vi "Validate Sequence File.vi"(8 "error in (no error)":errorcluster, 11 "Configured Steps In":T1[](array[typedef])) -> (0 "error out":errorcluster, 2 "Valid?":bool, 3 "Configured Steps Out":T1[](array[typedef]))   [LabVIEW 2018]
doc: "Compares the step names from the saved sequence file with the available steps. If one does not match, returns error 71."
uses:
  controls/Configured Step.ctl
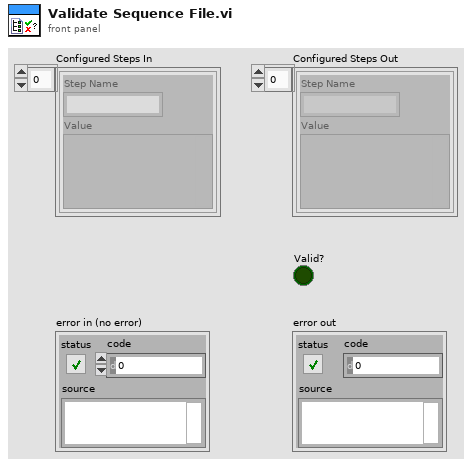
[diagram p1: front panel]
types:
  T1 = typedef "Configured Step.ctl" = cluster{"Step Name":string, "Value":variant}
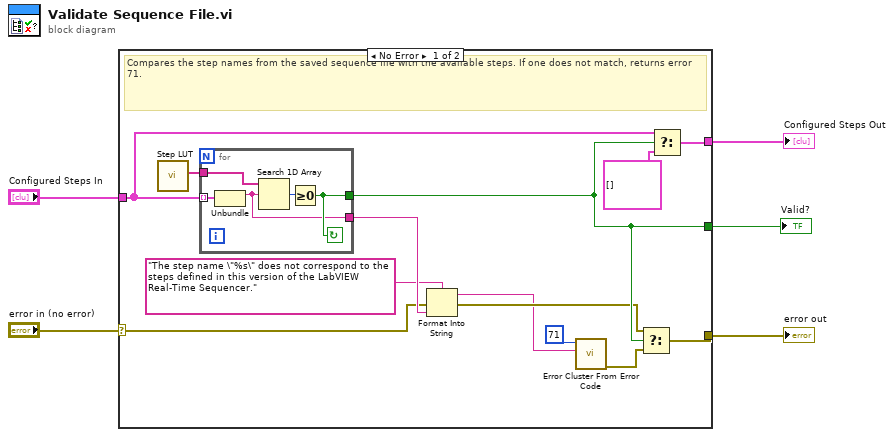
[diagram p0: block diagram]
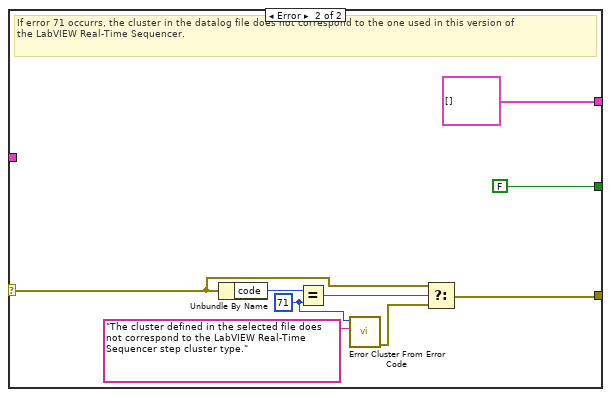
[diagram p2: hidden frame]
diagram:
  n1 = case shown="No Error" "error in (no error)" {
    selector: "error in (no error)" -> [w9 w25]
    tunnel: "Configured Steps In" -> [w14 _]
    tunnel: [w17 T1[] [] ("Configured Steps In")] -> w5
    tunnel: [w15 w24] -> w2
    tunnel: [w16 FALSE] -> w1
    frame No Error {
      # "Compares the step names from the saved sequence file with the available steps. If one does not match, returns error 71."
      n2 = call "Step LUT.vi"() -> ("Available Steps"=w18:string[])  [unwired: 10 in, 1 out]
      n3 = for {
        tunnel: w14 -> [w23] mode=indexing
        tunnel: w18 -> [w22]
        tunnel: [w20] -> w16
        tunnel: [w19] -> w10
        stop <- w20 continue-if-true
        n4 = Unbundle(w23) -> ("Step Name"=w19:string)  [unwired: 1 out]
        n5 = Search 1D Array(1D array=w22, element=w19) -> (index of element=w21:i32)  [unwired: 1 in]
        n6 = Greater Or Equal To 0?(x=w21) -> (x >= 0?=w20:bool)
      }
      n7 = Format Into String(format string="The step name \"%s\" does not correspond to the steps defined in this version of the LabVIEW Real-Time Sequencer." ("input 2"), error in=w9, w10) -> (resulting string=w7:string, error out=w8:errorcluster)  [unwired: 1 in]
      n8 = call <vilib>:"Error Cluster From Error Code.vi"("error message (\"\")"=w7, "error code (0)"=71 ("code")) -> ("error out"=w12:errorcluster)  [unwired: 7 in]
      n9 = Select(t=w8, s=w16, f=w12) -> (s? t:f=w15:errorcluster)
      n10 = Select(t=w14, s=w16, f=T1[] [] ("t")) -> (s? t:f=w17:T1[])
    }
    frame Error {
      w28 = 71 ("y")
      # "If error 71 occurrs, the cluster in the datalog file does not correspond to the one used in this version of\nthe LabVIEW Real-Time Sequencer."
      n11 = Unbundle By Name(w25) -> ("code"=w29:i32)
      n12 = Equal?(x=w29, y=w28) -> (x = y?=w32:bool)
      n13 = call <vilib>:"Error Cluster From Error Code.vi"("error message (\"\")"="The cluster defined in the selected file does not correspond to the LabVIEW Real-Time Sequencer step cluster type." ("error message (\"\")"), "error code (0)"=w28) -> ("error out"=w27:errorcluster)  [unwired: 7 in]
      n14 = Select(t=w25, s=w32, f=w27) -> (s? t:f=w24:errorcluster)
    }
  }
  "Configured Steps Out" <- w5
  "error out" <- w2
  "Valid?" <- w1
